vi "Main.vi"(9 "Marca":T1, 10 "Com Port":refnum<visa-resource-name>, 11 "Module Admin":refnum<class "Delacor_lib_QMH_Cloneable Module Admin.lvclass">) -> ()   [LabVIEW 2019, in "Multiple_uC.lvlib"]
doc: "This template is based off of the Queued Message Handler design pattern and the Queued Message Handler project template that ships with LabVIEW.\n\nThe main difference is that the queue is private to this module and communication between modules is performed via Broadcast and Request events.\n\nRequest events are wrapped in public API methods and are handled in the Event Handling Loop (EHL) of this VI. Any module can register for Broadcast events sent by this module. The EHL generates messages based on user interface actions.\n\nThe Message Handling Loop (MHL) processes messages generated by the EHL, or by other messages. The messages are string values, so new messages can be added easily to the Message Cases case structure in the MHL. Each message cluster can also provide an optional value for Message Data, which is a variant that can be converted to whatever message-specific data is required.\n_____\nBased on Delacor QMH Project Template 5.0.0.82."
uses:
  Multiple_uC.lvlib
  <vilib>/Delacor/Delacor QMH/Libraries/Cloneable Module Admin_class/Delacor_lib_QMH_Cloneable Module Admin.lvclass
  C:/Program Files/National Instruments/LabVIEW 2019/vi.lib/Delacor/Delacor QMH/Libraries/Module Admin_class/Delacor_lib_QMH_Module Admin.lvclass
  Clase Padre/Marca.ctl
  Module Data--cluster.ctl
  Clase Padre/Serial Device.lvclass
  <vilib>/Delacor/Delacor QMH/Libraries/Message Queue_class/Delacor_lib_QMH_Message Queue.lvclass/Delacor_lib_QMH_Message Queue.ctl
  <vilib>/Delacor/Delacor QMH/Libraries/Cloneable Module Admin_class/Delacor_lib_QMH_Cloneable Module Admin.lvclass/Delacor_lib_QMH_Cloneable Module Admin.ctl
  Stop Argument--cluster.ctl
  <vilib>/Delacor/Delacor QMH/Libraries/Module Admin_class/Delacor_lib_QMH_Module Admin.lvclass/Delacor_lib_QMH_Module Admin.ctl
  Write_1BIT Argument--cluster.ctl
  Write_1BIT (Reply Payload)--cluster.ctl
  Set 8 bits Argument--cluster.ctl
  Set 8 bits (Reply Payload)--cluster.ctl
  GET_1BIT Argument--cluster.ctl
  GET_1BIT (Reply Payload)--cluster.ctl
  GET_8BITS Argument--cluster.ctl
  GET_8BITS (Reply Payload)--cluster.ctl
  <vilib>/Utility/miscctls.llb/LVPointTypeDef.ctl
  Clases Hijos/NXP/NXP.lvclass
  C:/Users/Luis/Documents/Ingenieria/Git_versiones/PROYECTO-FINAL-INSTRUMENTACI-N-VIRTUAL/Clase Padre/Serial Device.lvclass
  Clases Hijos/Simulated/Simulated uC.lvclass
  Clases Hijos/Cypress/Cypress.lvclass
  Clase Padre/Serial Device.lvclass/Serial Device.ctl
  <vilib>/Delacor/Delacor QMH/Libraries/Message Queue_class/Delacor_lib_QMH_Enqueue Message (Single).vi
  <vilib>/Delacor/Delacor QMH/Libraries/Cloneable Module Admin_class/Delacor_lib_QMH_Get Module ID.vi
  <vilib>/Delacor/Delacor QMH/Libraries/Module Admin_class/Delacor_lib_QMH_Get External Launch.vi
  <vilib>/Utility/error.llb/Error Cluster From Error Code.vi
  <vilib>/ErrorRing/Error Ring.xnode
  <vilib>/Delacor/Delacor QMH/Libraries/Message Queue_class/Delacor_lib_QMH_Message Queue.lvclass
panel:
  in  "Read\n8 BITS":bool
  out "Response R 8BIT":string
  out "Response R 1BIT":string
  in  "GET 1BIT":u8 max=7
  out "Response W 8_B":string
  in  "Number":u8
  out "Response W1BIT":string
  in  "Encender\n W1BIT?":bool
  in  "Bit W1BIT":u8 max=7
  out "Response ADC":string
  in  "Channel adc":u8 max=9
  in  "Simulate MHL Error":bool
  in  "Simulate EHL Error":bool
  out "error out":errorcluster
  out "Status":string
  # "ADC"
  # "Write 1 Bit"
  # "Write 8 bit"
  # "Read 1 Bit"
  # "Read 8 bits"
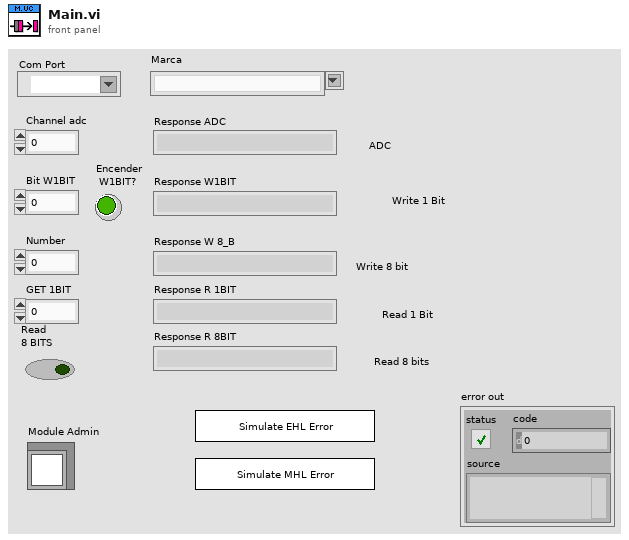
[diagram p1: front panel]
types:
  T1 = typedef "Marca.ctl" = string
  T2 = typedef "Multiple_uC.lvlib/Request Events--cluster.ctl" = cluster{"Stop Module":refnum<user-event>, "Show Panel":refnum<user-event>, "Hide Panel":refnum<user-event>, "Show Diagram":refnum<user-event>, "Get Module Execution Status":refnum<user-event>, "ADC´s View":refnum<user-event>, "Write_1BIT":refnum<user-event>, "Set 8 bits":refnum<user-event>, "GET_1BIT":refnum<user-event>, "GET_8BITS":refnum<user-event>}
  T3 = typedef "Multiple_uC.lvlib/Module Data--cluster.ctl" = cluster{"Status":string, "Serial Device.lvclass":refnum<class "Serial Device.lvclass">}
  T4 = enum32{"invalid lock state", "Not Locked", "Locked (No Password)", "Password-protected"}
  T5 = typedef "Multiple_uC.lvlib/Stop Argument--cluster.ctl" = cluster{"Module ID":i32, "Origin":string, "Exit via Stop Module Req?":bool, "Wait for Module to stop?":bool}
  T6 = typedef "Multiple_uC.lvlib/ADC´s View Argument--cluster.ctl" = cluster{"Module ID":i32, "Channel":u8, "Wait Notifier":refnum<notifier>, "wait for reply":bool}
  T7 = typedef "Multiple_uC.lvlib/Write_1BIT Argument--cluster.ctl" = cluster{"Module ID":i32, "Channel":u8, "Encender?":bool, "Wait Notifier":refnum<notifier>, "wait for reply":bool}
  T8 = typedef "Multiple_uC.lvlib/Set 8 bits Argument--cluster.ctl" = cluster{"Module ID":i32, "Number":u8, "Wait Notifier":refnum<notifier>, "wait for reply":bool}
  T9 = typedef "Multiple_uC.lvlib/GET_1BIT Argument--cluster.ctl" = cluster{"Module ID":i32, "GET 1BIT":u8, "Wait Notifier":refnum<notifier>, "wait for reply":bool}
  T10 = typedef "Multiple_uC.lvlib/GET_8BITS Argument--cluster.ctl" = cluster{"Module ID":i32, "Wait Notifier":refnum<notifier>, "wait for reply":bool, "Canal":u8}
  T11 = typedef "LVPointTypeDef.ctl" = cluster{"Horizontal":i16, "Vertical":i16}
  T12 = enum32{"Invalid", "Standard", "Closed", "Hidden", "Minimized", "Maximized"}
  T13 = typedef "Multiple_uC.lvlib/ADC´s View (Reply Payload)--cluster.ctl" = cluster{"Expected Response":string, "Numeric":dbl, "ADC´s View_error":errorcluster}
  T14 = typedef "Multiple_uC.lvlib/Write_1BIT (Reply Payload)--cluster.ctl" = cluster{"Response Write_1B":string, "Write_1BIT_error":errorcluster}
  T15 = typedef "Multiple_uC.lvlib/Set 8 bits (Reply Payload)--cluster.ctl" = cluster{"Response":string, "Set 8 bits_error":errorcluster}
  T16 = typedef "Multiple_uC.lvlib/GET_1BIT (Reply Payload)--cluster.ctl" = cluster{"Response 1BIT":string, "GET_1BIT_error":errorcluster}
  T17 = typedef "Multiple_uC.lvlib/GET_8BITS (Reply Payload)--cluster.ctl" = cluster{"Response 8Bits":string, "GET_8BITS_error":errorcluster}
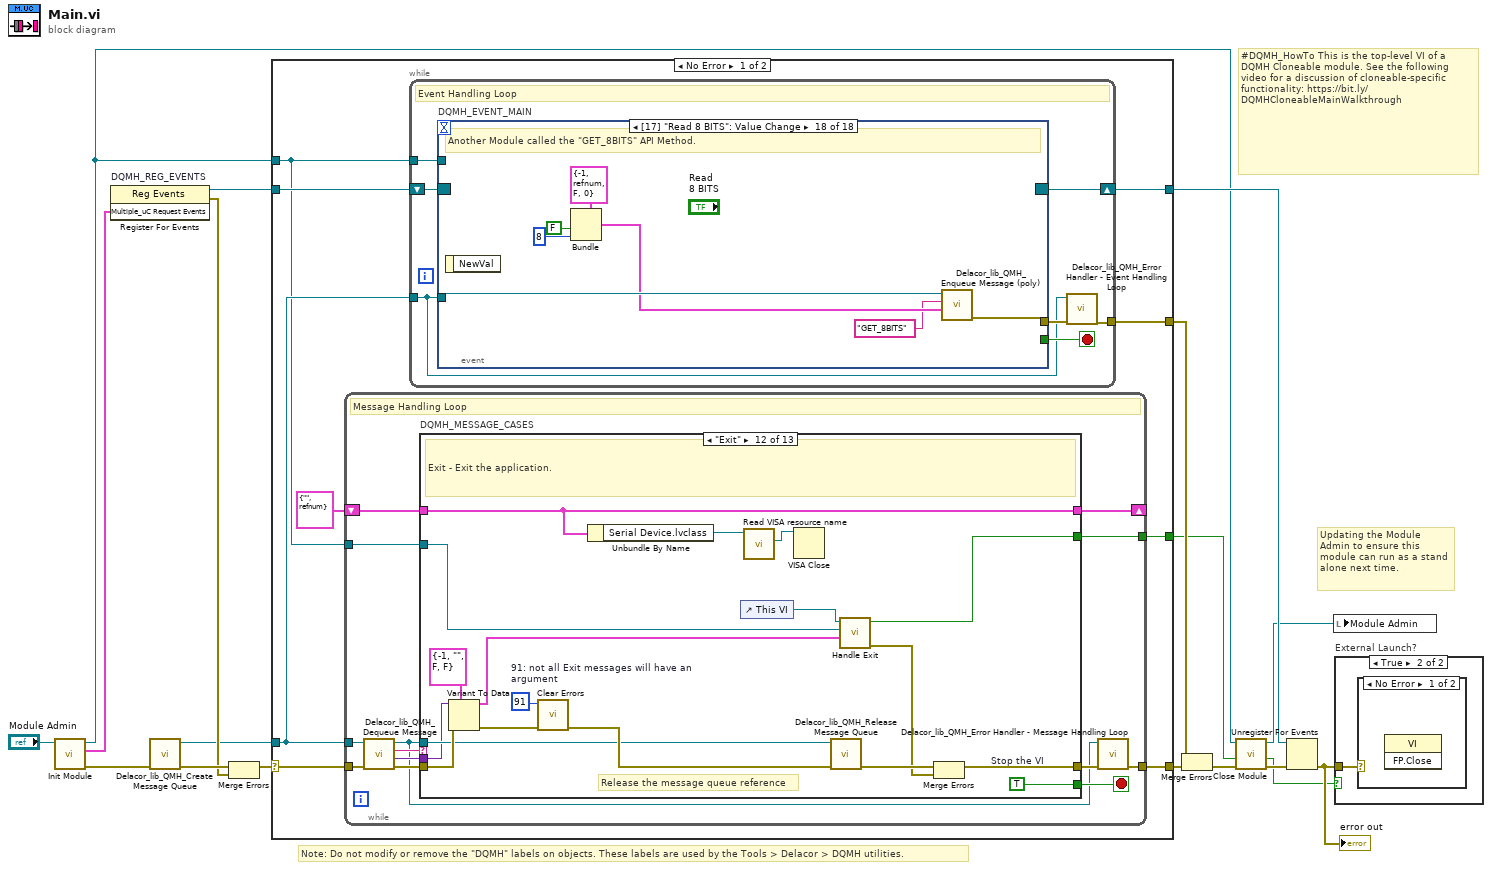
[diagram p0: block diagram]
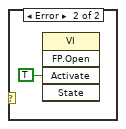
[diagram p3: hidden frame]
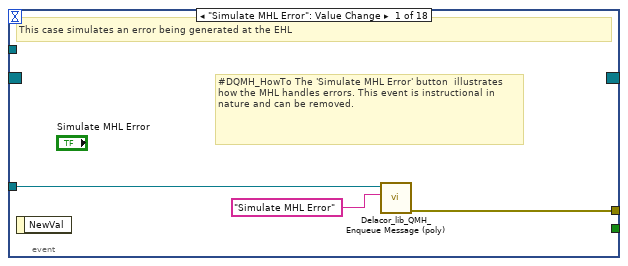
[diagram p4: hidden frame]
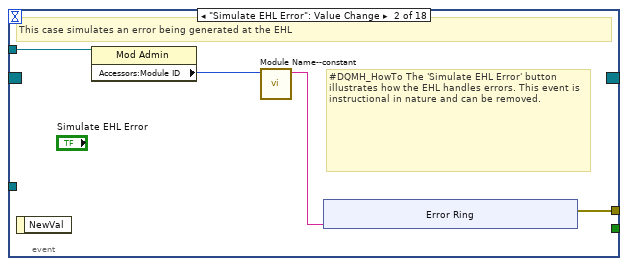
[diagram p5: hidden frame]
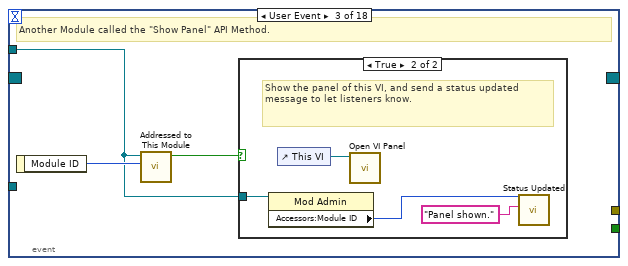
[diagram p6: hidden frame]
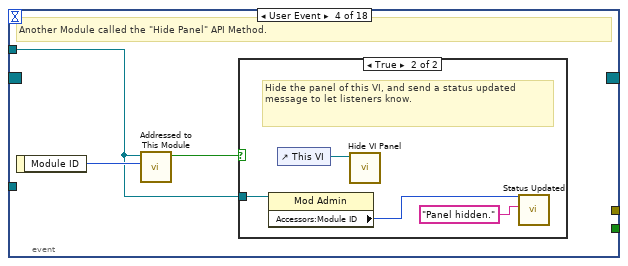
[diagram p8: hidden frame]
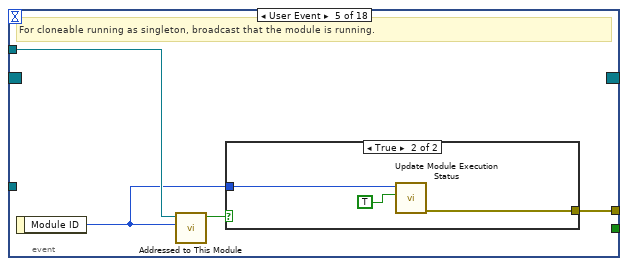
[diagram p10: hidden frame]
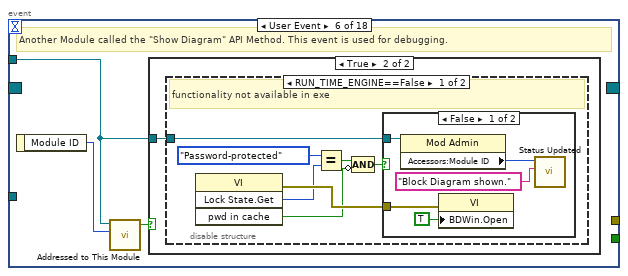
[diagram p12: hidden frame]
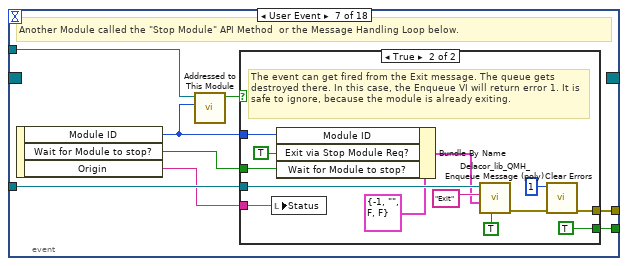
[diagram p16: hidden frame]
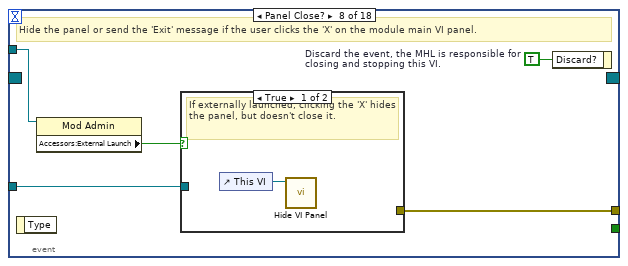
[diagram p18: hidden frame]
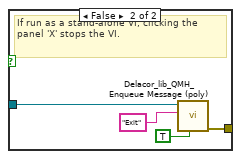
[diagram p19: hidden frame]
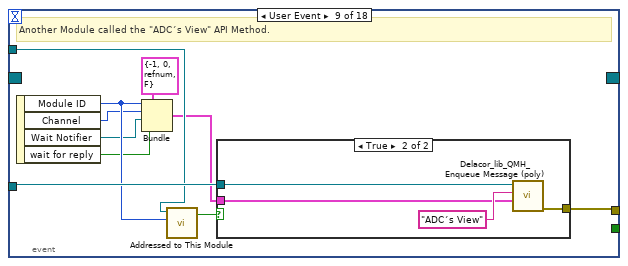
[diagram p20: hidden frame]
diagram:
  # "#DQMH_HowTo This is the top-level VI of a DQMH Cloneable module. See the following video for a discussion of cloneable-specific functionality: https://bit.ly/DQMHCloneableMainWalkthrough"
  # "Note: Do not modify or remove the \"DQMH\" labels on objects. These labels are used by the Tools > Delacor > DQMH utilities."
  # "Updating the Module Admin to ensure this module can run as a stand alone next time."
  n1 = call "Init Module.vi"("Cloneable Module Admin in"="Module Admin") -> ("error out"=w15:errorcluster, "Multiple_uC Request Events"=w7:T2, "Cloneable Module Admin out"=w4:refnum<class "Delacor_lib_QMH_Cloneable Module Admin.lvclass">)  [unwired: 8 in]
  n2 = register-events "DQMH_REG_EVENTS"(w7) -> (reference out=w8:refnum<event-registration>, error out=w10:errorcluster)  [unwired: 2 in]
  n3 = call <vilib>:"Delacor_lib_QMH_Create Message Queue.vi"("error in (no error)"=w15) -> ("error out"=w12:errorcluster, "Message Queue"=w6:refnum<class "Delacor_lib_QMH_Message Queue.lvclass">)  [unwired: 9 in]
  n4 = Merge Errors(w12, w10) -> (w11:errorcluster)
  n5 = case shown="No Error" w11 {
    selector: w11 -> [w25 w445]
    tunnel: [w27 w444] -> w16
    tunnel: [w24 w452] -> w9
    tunnel: w8 -> [w22 w452]
    tunnel: w6 -> [w21 w443]
    tunnel: [w26 _] -> w17
    tunnel: w4 -> [w20 w448]
    tunnel: [w19 _] -> w2
    frame No Error {
      n6 = while {
        tunnel: w21 -> [w227]
        shift-right: [w231] -> _
        shift-left: T3 {"Status"="", "Serial Device.lvclass"=refnum} ("Data Cluster") -> [w232]
        tunnel: w25 -> [w235]
        tunnel: [w233] -> w27
        tunnel: w20 -> [w225]
        tunnel: [w224] -> w19
        stop <- w230 stop-if-true
        # "Message Handling Loop"
        n7 = call-dynamic "Delacor_lib_QMH_Dequeue Message.vi"("error in (no error)"=w235, "Message Queue in"=w227) -> ("error out"=w234:errorcluster, "Message Data"=w228:variant, "Message"=w229:string, "Message Queue out"=w226:refnum<class "Delacor_lib_QMH_Message Queue.lvclass">)  [unwired: 6 in]
        n8 = case "DQMH_MESSAGE_CASES" shown="\"Exit\"" w229 {
          selector: w229 -> [_ _ _ _ _ _ _ _ _ _ _ _ w430]
          tunnel: w226 -> [_ _ _ _ _ _ _ _ _ w368 _ w420 _]
          tunnel: w234 -> [w262 w272 w288 w306 w323 w340 w357 w362 w364 w376 w401 w426 w432]
          tunnel: [w260 w272 w279 w297 w314 w331 w348 w361 w364 w372 w400 w423 w433] -> w236
          tunnel: w232 -> [w253 w271 w278 w296 w313 w330 w347 w360 w363 w365 w398 w410 w431]
          tunnel: [w252 w271 w278 w296 w313 w330 w347 w360 w363 w365 w398 w410 w431] -> w231
          tunnel: [_ _ _ _ _ _ _ _ _ _ _ w419 _] -> w230
          tunnel: w228 -> [_ _ w286 w304 w321 w338 w355 _ _ w371 _ w417 _]
          tunnel: w225 -> [w247 _ _ _ _ _ _ _ _ w370 w396 w413 w428]
          tunnel: [_ _ _ _ _ _ _ _ _ _ _ w415 _] -> w224
          frame "Initialize" {
            w244 = "Initial Message" ("Initial Message")
            # "Initialize - Any operation that needs to be done before the module can receive messages. Synchronize Caller Events.vi will inform Start Module.vi that the module has launched and is ready to receive messages. Module Did Init.vi will broadcast that the module initialized."
            n9 = call "Synchronize Caller Events.vi"("error in (no error)"=w262, "Module Admin"=w247) -> ("error out"=w261:errorcluster, "Module Admin out"=w246:refnum<class "Delacor_lib_QMH_Cloneable Module Admin.lvclass">)  [unwired: 8 in]
            n10 = property class="Mod Admin"(reference=w246) -> ("Accessors:Module ID"=w249:i32, "Accessors:External Launch"=w248:bool)  [unwired: 1 in, 2 out]
            n11 = case shown="\"N\", Default" "Marca" {
              tunnel: [refnum<class "NXP.lvclass"> refnum ("NXP.lvclass") refnum<class "Simulated uC.lvclass"> refnum ("Simulated uC.lvclass") refnum<class "Cypress.lvclass"> refnum ("Cypress.lvclass")] -> w243
              frame "N", Default {
                n12 = One Button Dialog(message="NXP") -> ()  [unwired: 1 in, 1 out]
              }
              frame "S" {
                n13 = One Button Dialog(message="Sim") -> ()  [unwired: 1 in, 1 out]
              }
              frame "C" {
                n14 = One Button Dialog(message="Cypress") -> ()  [unwired: 1 in, 1 out]
              }
            }
            n15 = call "Module Name--constant.vi"("Module ID"=w249) -> ("Module Name"=w257:string)  [unwired: 10 in]
            n16 = VISA Open(VISA resource name="Com Port") -> (VISA resource name=w238:refnum<visa-resource-name>)  [unwired: 4 in, 1 out]
            n17 = call "Write Marca.vi"("Marca"="Marca", "Serial Device in"=w243) -> ("Serial Device out"=w242:refnum<class "Serial Device.lvclass">)  [unwired: 8 in, 1 out]
            n18 = call "Write VISA resource name.vi"("VISA resource name"=w238, "Serial Device in"=w242) -> ("Serial Device out"=w240:refnum<class "Serial Device.lvclass">)  [unwired: 8 in, 1 out]
            n19 = property class="VI"("Front Panel.Title"=w257) -> (reference out=w259:refnum<vi>, error out=w264:errorcluster)  [unwired: 2 in]
            n20 = Select(t=T12."Hidden" ("State"), s=w248, f=T12."Standard" ("State")) -> (s? t:f=w254:T12)
            n21 = call-dynamic "Initialize.vi"("Serial Device in"=w240) -> ("Serial Device out"=w239:refnum<class "Serial Device.lvclass">)  [unwired: 9 in, 1 out]
            n22 = Bundle By Name(cluster=w253, "Serial Device.lvclass"=w239, "Status"=w244) -> (w252:T3)
            n23 = invoke class="VI" method="FP.Open"(reference=w259, error in=w264, "State"=w254) -> (reference out=w258:refnum<vi>, error out=w263:errorcluster)  [unwired: 2 in, 3 out]
            n24 = call "Module Name--constant.vi"("Module ID"=w249) -> ("Module Name"=w250:string)  [unwired: 10 in]
            n25 = invoke class="VI" method="FP.Center"(reference=w258, error in=w263) -> ()  [unwired: 1 in, 3 out]
            n26 = property on="Pane" class="Pane"("Origin"=T11 {"Horizontal"=0, "Vertical"=0}) -> ()  [unwired: 2 in, 2 out]
            n27 = call "Module Did Init.vi"("error in (no error)"=w261, "Initialized?"=TRUE, "Origin"=w250, "Module ID"=w249) -> ("error out"=w260:errorcluster)  [unwired: 7 in]
            "Status" <- w244
          }
          frame "--- Module Specific ---" {
            # "Separator -- The following cases handle messages specific to this Module."
          }
          frame "ADC´s View" {
            # "Request and wait for reply of ADC Channel"
            n28 = Unbundle By Name(w278) -> ("Serial Device.lvclass"=w277:refnum<class "Serial Device.lvclass">)
            n29 = Variant To Data(error in=w288, type=T6 {"Module ID"=-1, "Channel"=0, "Wait Notifier"=refnum, "wait for reply"=FALSE} ("ADC´s View Argument"), Variant=w286) -> (data=w284:T6, error out=w287:errorcluster)
            n30 = Unbundle By Name(w284) -> ("Channel"=w276:u8, "Wait Notifier"=w283:refnum<notifier>, "wait for reply"=w282:bool)
            n31 = call-dynamic "Send_ADC.vi"("Channel"=w276, "Serial Device in"=w277) -> ("error out"=w273:errorcluster, "Response"=w274:string)  [unwired: 7 in, 1 out]
            "Response ADC" <- w274
            n32 = Decimal String To Number(string=w274) -> (offset past number=w275:i32)  [unwired: 2 in, 1 out]
            n33 = Bundle By Name(cluster=T13 {"Expected Response"="", "Numeric"=0.0, "ADC´s View_error"={"status"=FALSE, "code"=0, "source"=""}} ("ADC´s View (Reply Payload)"), "Expected Response"=w274, "Numeric"=w275, "ADC´s View_error"=w273) -> (w281:T13)
            n34 = case shown="True" w282 {
              tunnel: w283 -> [_ w290]
              tunnel: w281 -> [_ w289]
              frame False {
              }
              frame True {
                n35 = Send Notification(notification=w289, notifier=w290) -> ()  [unwired: 1 in, 2 out]
              }
            }
            n36 = Merge Errors(w287, w273) -> (w279:errorcluster)
          }
          frame "Write_1BIT" {
            # "Event to rewrite the value of one bit in an array"
            n37 = Unbundle By Name(w296) -> ("Serial Device.lvclass"=w295:refnum<class "Serial Device.lvclass">)
            n38 = Variant To Data(error in=w306, type=T7 {"Module ID"=-1, "Channel"=0, "Encender?"=FALSE, "Wait Notifier"=refnum, "wait for reply"=FALSE} ("Write_1BIT Argument"), Variant=w304) -> (data=w302:T7, error out=w305:errorcluster)
            n39 = Unbundle By Name(w302) -> ("Channel"=w294:u8, "Encender?"=w293:bool, "Wait Notifier"=w301:refnum<notifier>, "wait for reply"=w300:bool)
            n40 = call-dynamic "Send_SET_1BIT.vi"("Encender?"=w293, "Channel"=w294, "Serial Device in"=w295) -> ("error out"=w291:errorcluster, "Response"=w292:string)  [unwired: 6 in, 1 out]
            "Response W1BIT" <- w292
            n41 = Bundle By Name(cluster=T14 {"Response Write_1B"="", "Write_1BIT_error"={"status"=FALSE, "code"=0, "source"=""}} ("Write_1BIT (Reply Payload)"), "Response Write_1B"=w292, "Write_1BIT_error"=w291) -> (w299:T14)
            n42 = case shown="True" w300 {
              tunnel: w301 -> [_ w308]
              tunnel: w299 -> [_ w307]
              frame False {
              }
              frame True {
                n43 = Send Notification(notification=w307, notifier=w308) -> ()  [unwired: 1 in, 2 out]
              }
            }
            n44 = Merge Errors(w305, w291) -> (w297:errorcluster)
          }
          frame "Set 8 bits" {
            # "Set a number of 8 bits in the microcontroller"
            n45 = Unbundle By Name(w313) -> ("Serial Device.lvclass"=w309:refnum<class "Serial Device.lvclass">)
            n46 = Variant To Data(error in=w323, type=T8 {"Module ID"=-1, "Number"=0, "Wait Notifier"=refnum, "wait for reply"=FALSE} ("Set 8 bits Argument"), Variant=w321) -> (data=w319:T8, error out=w322:errorcluster)
            n47 = Unbundle By Name(w319) -> ("Number"=w312:u8, "Wait Notifier"=w318:refnum<notifier>, "wait for reply"=w317:bool)
            n48 = call-dynamic "Send_SET_8Bits.vi"("Channel"=w312, "Serial Device in"=w309) -> ("error out"=w310:errorcluster, "Response"=w311:string)  [unwired: 7 in, 1 out]
            "Response W 8_B" <- w311
            n49 = Bundle By Name(cluster=T15 {"Response"="", "Set 8 bits_error"={"status"=FALSE, "code"=0, "source"=""}} ("Set 8 bits (Reply Payload)"), "Response"=w311, "Set 8 bits_error"=w310) -> (w316:T15)
            n50 = case shown="False" w317 {
              tunnel: w318 -> [_ w325]
              tunnel: w316 -> [_ w324]
              frame False {
              }
              frame True {
                n51 = Send Notification(notification=w324, notifier=w325) -> ()  [unwired: 1 in, 2 out]
              }
            }
            n52 = Merge Errors(w322, w310) -> (w314:errorcluster)
          }
          frame "GET_1BIT" {
            # "Obtain the value of 1 specific bit of the input of the microcontroller"
            n53 = Unbundle By Name(w330) -> ("Serial Device.lvclass"=w329:refnum<class "Serial Device.lvclass">)
            n54 = Variant To Data(error in=w340, type=T9 {"Module ID"=-1, "GET 1BIT"=0, "Wait Notifier"=refnum, "wait for reply"=FALSE} ("GET_1BIT Argument"), Variant=w338) -> (data=w336:T9, error out=w339:errorcluster)
            n55 = Unbundle By Name(w336) -> ("GET 1BIT"=w328:u8, "Wait Notifier"=w335:refnum<notifier>, "wait for reply"=w334:bool)
            n56 = call-dynamic "Send_Get_1Bit.vi"("Channel"=w328, "Serial Device in"=w329) -> ("error out"=w326:errorcluster, "Response"=w327:string)  [unwired: 7 in, 1 out]
            "Response R 1BIT" <- w327
            n57 = Bundle By Name(cluster=T16 {"Response 1BIT"="", "GET_1BIT_error"={"status"=FALSE, "code"=0, "source"=""}} ("GET_1BIT (Reply Payload)"), "Response 1BIT"=w327, "GET_1BIT_error"=w326) -> (w333:T16)
            n58 = case shown="True" w334 {
              tunnel: w335 -> [_ w342]
              tunnel: w333 -> [_ w341]
              frame False {
              }
              frame True {
                n59 = Send Notification(notification=w341, notifier=w342) -> ()  [unwired: 1 in, 2 out]
              }
            }
            n60 = Merge Errors(w339, w326) -> (w331:errorcluster)
          }
          frame "GET_8BITS" {
            # "Event created to get the eight bits of the eight inputs in the microcontroller"
            n61 = Unbundle By Name(w347) -> ("Serial Device.lvclass"=w346:refnum<class "Serial Device.lvclass">)
            n62 = Variant To Data(error in=w357, type=T10 {"Module ID"=-1, "Wait Notifier"=refnum, "wait for reply"=FALSE, "Canal"=0} ("GET_8BITS Argument"), Variant=w355) -> (data=w353:T10, error out=w356:errorcluster)
            n63 = Unbundle By Name(w353) -> ("Canal"=w345:u8, "Wait Notifier"=w352:refnum<notifier>, "wait for reply"=w351:bool)
            n64 = call-dynamic "Send_Get_8Bits.vi"("Channel"=w345, "Serial Device in"=w346) -> ("error out"=w343:errorcluster, "Response"=w344:string)  [unwired: 7 in, 1 out]
            "Response R 8BIT" <- w344
            n65 = Bundle By Name(cluster=T17 {"Response 8Bits"="", "GET_8BITS_error"={"status"=FALSE, "code"=0, "source"=""}} ("GET_8BITS (Reply Payload)"), "Response 8Bits"=w344, "GET_8BITS_error"=w343) -> (w350:T17)
            n66 = case shown="True" w351 {
              tunnel: w352 -> [_ w359]
              tunnel: w350 -> [_ w358]
              frame False {
              }
              frame True {
                n67 = Send Notification(notification=w358, notifier=w359) -> ()  [unwired: 1 in, 2 out]
              }
            }
            n68 = Merge Errors(w356, w343) -> (w348:errorcluster)
          }
          frame "---Copy This Frame---" {
            # "Duplicate this frame when creating new messages.  Change this comment in the duplicated frame to describe this message."
            n69 = Merge Errors(w362) -> (w361:errorcluster)
          }
          frame "--- Exit and Error Handling---" {
            # "Separator - the following cases handle errors and exit messages."
          }
          frame "Error" {
            # "Error - Check the error message data and respond accordingly. This message is sent by the \"Error Handler\" VIs at the end of each loop in this application."
            n70 = property class="Mod Admin"(reference=w370) -> ("Accessors:External Launch"=w369:bool, "Accessors:Module ID"=w366:i32)  [unwired: 1 in, 2 out]
            n71 = Variant To Data(error in=w376, type=errorcluster {"status"=FALSE, "code"=0, "source"=""} ("error constant"), Variant=w371) -> (data=w377:errorcluster, error out=w374:errorcluster)
            n72 = call "Module Name--constant.vi"("Module ID"=w366) -> ("Module Name"=w367:string)  [unwired: 10 in]
            n73 = call "Error Reported.vi"("Additional Information"=w367, "Error"=w377, "Module ID"=w366) -> ()  [unwired: 8 in, 1 out]
            n74 = case shown="True" w369 {
              tunnel: [w382 w383] -> w373
              tunnel: w368 -> [w380 w384]
              tunnel: w377 -> [w381 w386]
              frame False {
                # "If the module is running standalone, then pop up an error dialog and call the \"Exit\" message."
                n75 = call <vilib>:"Simple Error Handler.vi"("error in (no error)"=w381) -> ()  [unwired: 4 in, 5 out]
                n76 = call-poly <vilib>:"Delacor_lib_QMH_Enqueue Message (poly).vi"("Priority Message? (F)"=TRUE, "Message"="Exit", "Message Queue in"=w380) -> ("error out"=w382:errorcluster)  [unwired: 7 in, 1 out]
              }
              frame True {
                n77 = Unbundle By Name(w386) -> ("code"=w385:i32)
                n78 = case shown="-1073807360" w385 {
                  tunnel: w384 -> [_ w390 w394]
                  tunnel: [_ w387 w391] -> w383
                  frame 0, Default {
                  }
                  frame -1073807360 {
                    n79 = call-poly <vilib>:"Delacor_lib_QMH_Enqueue Message (poly).vi"("Message"="Exit", "Message Queue in"=w390) -> ("error out"=w387:errorcluster)  [unwired: 8 in, 1 out]
                    n80 = One Button Dialog(message="Microcontrolador\nDesconectado\n:(\n\nFavor de revisar la conexión y vuelva a intentar") -> ()  [unwired: 1 in, 1 out]
                  }
                  frame -1073807343 {
                    n81 = One Button Dialog(message="Microcontrolador\nDesconectado\n:(\n\nFavor de revisar la conexión y vuelva a intentar") -> ()  [unwired: 1 in, 1 out]
                    n82 = call-poly <vilib>:"Delacor_lib_QMH_Enqueue Message (poly).vi"("Message"="Exit", "Message Queue in"=w394) -> ("error out"=w391:errorcluster)  [unwired: 8 in, 1 out]
                  }
                }
              }
            }
            n83 = Merge Errors(w374, w373) -> (w372:errorcluster)
            n84 = local write "error out"(w372) -> ()
          }
          frame "Simulate MHL Error" {
            # "#DQMH_HowTo The 'Simulate MHL Error' button  illustrates how the MHL handles errors. This event is instructional in nature and can be removed."
            # "Simulate an error occurring at the MHL"
            n85 = property class="Mod Admin"(reference=w396) -> ("Accessors:Module ID"=w397:i32)  [unwired: 1 in, 2 out]
            n86 = call "Module Name--constant.vi"("Module ID"=w397) -> ("Module Name"=w395:string)  [unwired: 10 in]
            n87 = xnode "Error Ring"("parameter 0"=w395) -> ("error out"=w399:errorcluster)
            n88 = Merge Errors(w401, w399) -> (w400:errorcluster)
          }
          frame "Exit" {
            w418 = 91  # 91: not all Exit messages will have an argument
            w419 = TRUE  # Stop the VI
            # "Release the message queue reference"
            # "Exit - Exit the application."
            n89 = Variant To Data(error in=w426, type=T5 {"Module ID"=-1, "Origin"="", "Exit via Stop Module Req?"=FALSE, "Wait for Module to stop?"=FALSE} ("Stop Argument"), Variant=w417) -> (data=w414:T5, error out=w421:errorcluster)
            n90 = call <vilib>:"Clear Errors.vi"("error in (no error)"=w421, "specific error code to clear (0: all)"=w418) -> ("error out"=w425:errorcluster)  [unwired: 4 in, 1 out]
            n91 = Unbundle By Name(w410) -> ("Serial Device.lvclass"=w409:refnum<class "Serial Device.lvclass">)
            n92 = control-ref of="This VI"() -> (w412:refnum<vi>)
            n93 = call "Read VISA resource name.vi"("Serial Device in"=w409) -> ("VISA resource name"=w411:refnum<visa-resource-name>)  [unwired: 8 in, 2 out]
            n94 = VISA Close(VISA resource name=w411) -> ()  [unwired: 1 in, 1 out]
            n95 = call-dynamic "Delacor_lib_QMH_Release Message Queue.vi"("error in (no error)"=w425, "Message Queue"=w420) -> ("error out"=w424:errorcluster)  [unwired: 9 in]
            n96 = call "Handle Exit.vi"("Stop Argument"=w414, "Module Admin in"=w413, "VI reference"=w412) -> ("error out"=w422:errorcluster, "Wait for Stop?"=w415:bool)  [unwired: 7 in]
            n97 = Merge Errors(w424, w422) -> (w423:errorcluster)
          }
          frame Default {
            # "'Default' case only runs if there is a message that isn't defined in any of the other cases.  Output a programming error."
            n98 = property class="Mod Admin"(reference=w428) -> ("Accessors:Module ID"=w427:i32)  [unwired: 1 in, 2 out]
            n99 = call "Module Name--constant.vi"("Module ID"=w427) -> ("Module Name"=w429:string)  [unwired: 10 in]
            n100 = xnode "Error Ring"("parameter 0"=w430, "parameter 1"=w429) -> ("error out"=w434:errorcluster)
            n101 = Merge Errors(w432, w434) -> (w433:errorcluster)
          }
        }
        n102 = call-dynamic "Delacor_lib_QMH_Error Handler - Message Handling Loop.vi"("error in (no error)"=w236, "Message Queue in"=w226) -> ("dup error in"=w233:errorcluster)  [unwired: 8 in, 1 out]
      }
      n103 = while {
        tunnel: w21 -> [w28]
        shift-right: [w31] -> w24
        shift-left: w22 -> [w32]
        tunnel: [w33] -> w26
        tunnel: w20 -> [w29]
        stop <- w30 stop-if-true
        # "Event Handling Loop"
        n104 = event "DQMH_EVENT_MAIN" shown="[17] \"Read 8 BITS\": Value Change" {
          selector: w32 -> [_ _ _ _ _ _ _ _ _ _ _ _ _ _ _ _ _ _]
          dyn-events: [_ _ _ _ _ _ _ _ _ _ _ _ _ _ _ _ _ _] -> w31
          timeout: _ -> [_ _ _ _ _ _ _ _ _ _ _ _ _ _ _ _ _ _]
          tunnel: [_ _ _ _ _ _ w89 _ _ _ _ _ _ _ _ _ _ _] -> w30
          tunnel: w28 -> [w36 _ _ _ _ _ w92 w108 w126 w137 w148 w160 w170 w181 w191 w202 w212 w223]
          tunnel: [w37 w41 _ _ w66 _ w93 w111 w117 w134 w138 w157 w161 w178 w182 w199 w206 w220] -> w34
          tunnel: w29 -> [_ w40 w49 w56 w64 w70 w91 w109 w124 _ w146 _ w168 _ w189 _ w210 _]
          event "Simulate MHL Error": Value Change {
            # "#DQMH_HowTo The 'Simulate MHL Error' button  illustrates how the MHL handles errors. This event is instructional in nature and can be removed."
            # "This case simulates an error being generated at the EHL"
            n105 = event-data() -> ()  [unwired: 1 in, 1 out]
            n106 = call-poly <vilib>:"Delacor_lib_QMH_Enqueue Message (poly).vi"("Message"="Simulate MHL Error", "Message Queue in"=w36) -> ("error out"=w37:errorcluster)  [unwired: 8 in, 1 out]
          }
          event "Simulate EHL Error": Value Change {
            # "#DQMH_HowTo The 'Simulate EHL Error' button  illustrates how the EHL handles errors. This event is instructional in nature and can be removed."
            # "This case simulates an error being generated at the EHL"
            n107 = event-data() -> ()  [unwired: 1 in, 1 out]
            n108 = property class="Mod Admin"(reference=w40) -> ("Accessors:Module ID"=w39:i32)  [unwired: 1 in, 2 out]
            n109 = call "Module Name--constant.vi"("Module ID"=w39) -> ("Module Name"=w38:string)  [unwired: 10 in]
            n110 = xnode "Error Ring"("parameter 0"=w38) -> ("error out"=w41:errorcluster)
          }
          event User Event {
            # "Another Module called the \"Show Panel\" API Method."
            n111 = event-data() -> ("Module ID"=w50:i32)  [unwired: 1 in]
            n112 = call "Addressed to This Module.vi"("Module ID from Argument"=w50, "Module Admin"=w49) -> ("Addressed to this instance?"=w51:bool)  [unwired: 8 in, 1 out]
            n113 = case shown="True" w51 {
              tunnel: w49 -> [_ w53]
              frame False {
              }
              frame True {
                # "Show the panel of this VI, and send a status updated message to let listeners know."
                n114 = property class="Mod Admin"(reference=w53) -> ("Accessors:Module ID"=w52:i32)  [unwired: 1 in, 2 out]
                n115 = control-ref of="This VI"() -> (w55:refnum<vi>)
                n116 = call "Open VI Panel.vi"("VI"=w55) -> ()  [unwired: 10 in, 1 out]
                n117 = call "Status Updated.vi"("Status"="Panel shown." ("format string"), "Module ID"=w52) -> ()  [unwired: 9 in, 1 out]
              }
            }
          }
          event User Event {
            # "Another Module called the \"Hide Panel\" API Method."
            n118 = event-data() -> ("Module ID"=w57:i32)  [unwired: 1 in]
            n119 = call "Addressed to This Module.vi"("Module ID from Argument"=w57, "Module Admin"=w56) -> ("Addressed to this instance?"=w58:bool)  [unwired: 8 in, 1 out]
            n120 = case shown="True" w58 {
              tunnel: w56 -> [_ w60]
              frame False {
              }
              frame True {
                # "Hide the panel of this VI, and send a status updated message to let listeners know."
                n121 = property class="Mod Admin"(reference=w60) -> ("Accessors:Module ID"=w59:i32)  [unwired: 1 in, 2 out]
                n122 = control-ref of="This VI"() -> (w62:refnum<vi>)
                n123 = call "Hide VI Panel.vi"("VI"=w62) -> ()  [unwired: 10 in, 1 out]
                n124 = call "Status Updated.vi"("Status"="Panel hidden." ("format string"), "Module ID"=w59) -> ()  [unwired: 9 in, 1 out]
              }
            }
          }
          event User Event {
            # "For cloneable running as singleton, broadcast that the module is running."
            n125 = event-data() -> ("Module ID"=w63:i32)  [unwired: 1 in]
            n126 = call "Addressed to This Module.vi"("Module ID from Argument"=w63, "Module Admin"=w64) -> ("Addressed to this instance?"=w65:bool)  [unwired: 8 in, 1 out]
            n127 = case shown="True" w65 {
              tunnel: [_ w69] -> w66
              tunnel: w63 -> [_ w68]
              frame False {
              }
              frame True {
                n128 = call "Update Module Execution Status.vi"("Running?"=TRUE, "Module ID"=w68) -> ("error out"=w69:errorcluster)  [unwired: 9 in]
              }
            }
          }
          event User Event {
            # "Another Module called the \"Show Diagram\" API Method. This event is used for debugging."
            n129 = event-data() -> ("Module ID"=w71:i32)  [unwired: 1 in]
            n130 = call "Addressed to This Module.vi"("Module ID from Argument"=w71, "Module Admin"=w70) -> ("Addressed to this instance?"=w72:bool)  [unwired: 8 in, 1 out]
            n131 = case shown="True" w72 {
              tunnel: w70 -> [_ w73]
              frame False {
              }
              frame True {
                n132 = disable-structure shown="RUN_TIME_ENGINE==False" {
                  disable-tunnel: w73 -> [w74 _]
                  frame condition #0 (active) {
                    # "functionality not available in exe"
                    n133 = invoke class="VI" method="Lock State.Get"() -> (error out=w80:errorcluster, "Get Lock State"=w79:T4, "pwd in cache"=w76:bool)  [unwired: 4 in, 1 out]
                    n134 = Equal?(x=T4."Password-protected", y=w79) -> (x = y?=w77:bool)
                    n135 = Compound Arithmetic op=AND(w77, invert w76) -> (w75:bool)
                    n136 = case shown="False" w75 {
                      tunnel: w80 -> [w85 _]
                      tunnel: w74 -> [w82 _]
                      frame False {
                        n137 = property class="Mod Admin"(reference=w82) -> ("Accessors:Module ID"=w81:i32)  [unwired: 1 in, 2 out]
                        n138 = property class="VI"(error in=w85, "BDWin.Open"=TRUE ("Block Diagram Window:Open")) -> ()  [unwired: 1 in, 2 out]
                        n139 = call "Status Updated.vi"("Status"="Block Diagram shown." ("format string"), "Module ID"=w81) -> ()  [unwired: 9 in, 1 out]
                      }
                      frame True {
                        # "Password-protected VI, and the password is not in the cache. Do not show the diagram."
                      }
                    }
                  }
                  frame condition #1 {
                  }
                }
              }
            }
          }
          event User Event {
            # "Another Module called the \"Stop Module\" API Method  or the Message Handling Loop below."
            n140 = event-data() -> ("Module ID"=w87:i32, "Wait for Module to stop?"=w88:bool, "Origin"=w86:string)  [unwired: 1 in]
            n141 = call "Addressed to This Module.vi"("Module ID from Argument"=w87, "Module Admin"=w91) -> ("Addressed to this instance?"=w90:bool)  [unwired: 8 in, 1 out]
            n142 = case shown="True" w90 {
              tunnel: [_ w105] -> w93
              tunnel: w92 -> [_ w101]
              tunnel: [_ TRUE] -> w89
              tunnel: w88 -> [_ w96]
              tunnel: w87 -> [_ w98]
              tunnel: w86 -> [_ w94]
              frame False {
              }
              frame True {
                # "The event can get fired from the Exit message. The queue gets destroyed there. In this case, the Enqueue VI will return error 1. It is safe to ignore, because the module is already exiting."
                n143 = local write "Status"(w94) -> ()
                n144 = Bundle By Name(cluster=T5 {"Module ID"=-1, "Origin"="", "Exit via Stop Module Req?"=FALSE, "Wait for Module to stop?"=FALSE} ("Stop Argument"), "Module ID"=w98, "Exit via Stop Module Req?"=TRUE, "Wait for Module to stop?"=w96) -> (w95:T5)
                n145 = call-poly <vilib>:"Delacor_lib_QMH_Enqueue Message (poly).vi"("Priority Message? (F)"=TRUE, "Message Data"=w95, "Message"="Exit", "Message Queue in"=w101) -> ("error out"=w106:errorcluster)  [unwired: 6 in, 1 out]
                n146 = call <vilib>:"Clear Errors.vi"("error in (no error)"=w106, "specific error code to clear (0: all)"=1) -> ("error out"=w105:errorcluster)  [unwired: 4 in, 1 out]
              }
            }
          }
          event Panel Close? {
            w110 = TRUE  # Discard the event, the MHL is responsible for closing and stopping this VI.
            # "Hide the panel or send the 'Exit' message if the user clicks the 'X' on the module main VI panel."
            n147 = event-data() -> ()  [unwired: 1 in, 1 out]
            n148 = property class="Mod Admin"(reference=w109) -> ("Accessors:External Launch"=w107:bool)  [unwired: 1 in, 2 out]
            n149 = case shown="True" w107 {
              tunnel: w108 -> [_ w115]
              tunnel: [_ w116] -> w111
              frame True {
                # "If externally launched, clicking the 'X' hides the panel, but doesn't close it."
                n150 = control-ref of="This VI"() -> (w112:refnum<vi>)
                n151 = call "Hide VI Panel.vi"("VI"=w112) -> ()  [unwired: 10 in, 1 out]
              }
              frame False {
                # "If run as a stand-alone VI, clicking the panel 'X' stops the VI."
                n152 = call-poly <vilib>:"Delacor_lib_QMH_Enqueue Message (poly).vi"("Priority Message? (F)"=TRUE, "Message"="Exit", "Message Queue in"=w115) -> ("error out"=w116:errorcluster)  [unwired: 7 in, 1 out]
              }
            }
            n153 = event-data("Discard?"=w110) -> ()  [unwired: 1 in, 1 out]
          }
          event User Event {
            # "Another Module called the \"ADC´s View\" API Method."
            n154 = event-data() -> ("Module ID"=w121:i32, "Channel"=w120:u8, "Wait Notifier"=w119:refnum<notifier>, "wait for reply"=w118:bool)  [unwired: 1 in]
            n155 = Bundle(cluster=T6 {"Module ID"=-1, "Channel"=0, "Wait Notifier"=refnum, "wait for reply"=FALSE} ("ADC´s View Argument"), "Module ID"=w121, "Channel"=w120, "Wait Notifier"=w119, "wait for reply"=w118) -> (w122:T6)
            n156 = call "Addressed to This Module.vi"("Module ID from Argument"=w121, "Module Admin"=w124) -> ("Addressed to this instance?"=w125:bool)  [unwired: 8 in, 1 out]
            n157 = case shown="True" w125 {
              tunnel: w126 -> [_ w130]
              tunnel: w122 -> [_ w128]
              tunnel: [_ w127] -> w117
              frame False {
              }
              frame True {
                n158 = call-poly <vilib>:"Delacor_lib_QMH_Enqueue Message (poly).vi"("Message Data"=w128, "Message"="ADC´s View", "Message Queue in"=w130) -> ("error out"=w127:errorcluster)  [unwired: 7 in, 1 out]
              }
            }
          }
          event "Channel adc": Value Change {
            # "Local Channel ADC"
            n159 = event-data() -> ()  [unwired: 1 in, 3 out]
            n160 = Bundle(cluster=T6 {"Module ID"=-1, "Channel"=0, "Wait Notifier"=refnum, "wait for reply"=FALSE} ("ADC´s View Argument"), "Channel"="Channel adc", "wait for reply"=FALSE) -> (w135:T6)  [unwired: 2 in]
            n161 = call-poly <vilib>:"Delacor_lib_QMH_Enqueue Message (poly).vi"("Message Data"=w135, "Message"="ADC´s View", "Message Queue in"=w137) -> ("error out"=w134:errorcluster)  [unwired: 7 in, 1 out]
          }
          event User Event {
            # "Another Module called the \"Write_1BIT\" API Method."
            n162 = event-data() -> ("Module ID"=w143:i32, "Channel"=w142:u8, "Encender?"=w141:bool, "Wait Notifier"=w140:refnum<notifier>, "wait for reply"=w139:bool)  [unwired: 1 in]
            n163 = Bundle(cluster=T7 {"Module ID"=-1, "Channel"=0, "Encender?"=FALSE, "Wait Notifier"=refnum, "wait for reply"=FALSE} ("Write_1BIT Argument"), "Module ID"=w143, "Channel"=w142, "Encender?"=w141, "Wait Notifier"=w140, "wait for reply"=w139) -> (w144:T7)
            n164 = call "Addressed to This Module.vi"("Module ID from Argument"=w143, "Module Admin"=w146) -> ("Addressed to this instance?"=w147:bool)  [unwired: 8 in, 1 out]
            n165 = case shown="True" w147 {
              tunnel: w148 -> [_ w152]
              tunnel: w144 -> [_ w150]
              tunnel: [_ w149] -> w138
              frame False {
              }
              frame True {
                n166 = call-poly <vilib>:"Delacor_lib_QMH_Enqueue Message (poly).vi"("Message Data"=w150, "Message"="Write_1BIT", "Message Queue in"=w152) -> ("error out"=w149:errorcluster)  [unwired: 7 in, 1 out]
              }
            }
          }
          event "Bit W1BIT": Value Change {
            # "Another Module called the \"Write_1BIT\" API Method."
            n167 = event-data() -> ()  [unwired: 1 in, 1 out]
            n168 = Bundle(cluster=T7 {"Module ID"=-1, "Channel"=0, "Encender?"=FALSE, "Wait Notifier"=refnum, "wait for reply"=FALSE} ("Write_1BIT Argument"), "Channel"="Bit W1BIT", "Encender?"="Encender\n W1BIT?", "wait for reply"=FALSE) -> (w158:T7)  [unwired: 2 in]
            n169 = call-poly <vilib>:"Delacor_lib_QMH_Enqueue Message (poly).vi"("Message Data"=w158, "Message"="Write_1BIT", "Message Queue in"=w160) -> ("error out"=w157:errorcluster)  [unwired: 7 in, 1 out]
          }
          event User Event {
            # "Another Module called the \"Set 8 bits\" API Method."
            n170 = event-data() -> ("Module ID"=w165:i32, "Number"=w164:u8, "Wait Notifier"=w163:refnum<notifier>, "wait for reply"=w162:bool)  [unwired: 1 in]
            n171 = Bundle(cluster=T8 {"Module ID"=-1, "Number"=0, "Wait Notifier"=refnum, "wait for reply"=FALSE} ("Set 8 bits Argument"), "Module ID"=w165, "Number"=w164, "Wait Notifier"=w163, "wait for reply"=w162) -> (w166:T8)
            n172 = call "Addressed to This Module.vi"("Module ID from Argument"=w165, "Module Admin"=w168) -> ("Addressed to this instance?"=w169:bool)  [unwired: 8 in, 1 out]
            n173 = case shown="True" w169 {
              tunnel: w170 -> [_ w174]
              tunnel: w166 -> [_ w172]
              tunnel: [_ w171] -> w161
              frame False {
              }
              frame True {
                n174 = call-poly <vilib>:"Delacor_lib_QMH_Enqueue Message (poly).vi"("Message Data"=w172, "Message"="Set 8 bits", "Message Queue in"=w174) -> ("error out"=w171:errorcluster)  [unwired: 7 in, 1 out]
              }
            }
          }
          event "Number": Value Change {
            # "Another Module called the \"Set 8 bits\" API Method."
            n175 = event-data() -> ()  [unwired: 1 in, 1 out]
            n176 = Bundle(cluster=T8 {"Module ID"=-1, "Number"=0, "Wait Notifier"=refnum, "wait for reply"=FALSE} ("Set 8 bits Argument"), "Number"="Number", "wait for reply"=FALSE) -> (w179:T8)  [unwired: 2 in]
            n177 = call-poly <vilib>:"Delacor_lib_QMH_Enqueue Message (poly).vi"("Message Data"=w179, "Message"="Set 8 bits", "Message Queue in"=w181) -> ("error out"=w178:errorcluster)  [unwired: 7 in, 1 out]
          }
          event User Event {
            # "Another Module called the \"GET_1BIT\" API Method."
            n178 = event-data() -> ("Module ID"=w186:i32, "GET 1BIT"=w185:u8, "Wait Notifier"=w184:refnum<notifier>, "wait for reply"=w183:bool)  [unwired: 1 in]
            n179 = Bundle(cluster=T9 {"Module ID"=-1, "GET 1BIT"=0, "Wait Notifier"=refnum, "wait for reply"=FALSE} ("GET_1BIT Argument"), "Module ID"=w186, "GET 1BIT"=w185, "Wait Notifier"=w184, "wait for reply"=w183) -> (w187:T9)
            n180 = call "Addressed to This Module.vi"("Module ID from Argument"=w186, "Module Admin"=w189) -> ("Addressed to this instance?"=w190:bool)  [unwired: 8 in, 1 out]
            n181 = case shown="True" w190 {
              tunnel: w191 -> [_ w195]
              tunnel: w187 -> [_ w193]
              tunnel: [_ w192] -> w182
              frame False {
              }
              frame True {
                n182 = call-poly <vilib>:"Delacor_lib_QMH_Enqueue Message (poly).vi"("Message Data"=w193, "Message"="GET_1BIT", "Message Queue in"=w195) -> ("error out"=w192:errorcluster)  [unwired: 7 in, 1 out]
              }
            }
          }
          event "GET 1BIT": Value Change {
            # "Another Module called the \"GET_1BIT\" API Method."
            n183 = event-data() -> ()  [unwired: 1 in, 1 out]
            n184 = Bundle(cluster=T9 {"Module ID"=-1, "GET 1BIT"=0, "Wait Notifier"=refnum, "wait for reply"=FALSE} ("GET_1BIT Argument"), "GET 1BIT"="GET 1BIT", "wait for reply"=FALSE) -> (w200:T9)  [unwired: 2 in]
            n185 = call-poly <vilib>:"Delacor_lib_QMH_Enqueue Message (poly).vi"("Message Data"=w200, "Message"="GET_1BIT", "Message Queue in"=w202) -> ("error out"=w199:errorcluster)  [unwired: 7 in, 1 out]
          }
          event User Event {
            # "Another Module called the \"GET_8BITS\" API Method."
            n186 = event-data() -> ("Module ID"=w207:i32, "Canal"=w203:u8, "Wait Notifier"=w205:refnum<notifier>, "wait for reply"=w204:bool)  [unwired: 1 in]
            n187 = Bundle(cluster=T10 {"Module ID"=-1, "Wait Notifier"=refnum, "wait for reply"=FALSE, "Canal"=0} ("GET_8BITS Argument"), "Module ID"=w207, "Wait Notifier"=w205, "wait for reply"=w204, "Canal"=w203) -> (w208:T10)
            n188 = call "Addressed to This Module.vi"("Module ID from Argument"=w207, "Module Admin"=w210) -> ("Addressed to this instance?"=w211:bool)  [unwired: 8 in, 1 out]
            n189 = case shown="True" w211 {
              tunnel: w212 -> [_ w216]
              tunnel: w208 -> [_ w214]
              tunnel: [_ w213] -> w206
              frame False {
              }
              frame True {
                n190 = call-poly <vilib>:"Delacor_lib_QMH_Enqueue Message (poly).vi"("Message Data"=w214, "Message"="GET_8BITS", "Message Queue in"=w216) -> ("error out"=w213:errorcluster)  [unwired: 7 in, 1 out]
              }
            }
          }
          event "Read\n8 BITS": Value Change {
            # "Another Module called the \"GET_8BITS\" API Method."
            n191 = event-data() -> ()  [unwired: 1 in, 1 out]
            n192 = Bundle(cluster=T10 {"Module ID"=-1, "Wait Notifier"=refnum, "wait for reply"=FALSE, "Canal"=0} ("GET_8BITS Argument"), "wait for reply"=FALSE, "Canal"=u8 8) -> (w221:T10)  [unwired: 2 in]
            n193 = call-poly <vilib>:"Delacor_lib_QMH_Enqueue Message (poly).vi"("Message Data"=w221, "Message"="GET_8BITS", "Message Queue in"=w223) -> ("error out"=w220:errorcluster)  [unwired: 7 in, 1 out]
          }
        }
        n194 = call-dynamic "Delacor_lib_QMH_Error Handler - Event Handling Loop.vi"("error in (no error)"=w34, "Message Queue in"=w28) -> ("dup error in"=w33:errorcluster)  [unwired: 8 in, 1 out]
      }
    }
    frame Error {
      n195 = call "Synchronize Caller Events.vi"("Module Admin"=w448) -> ("Module Admin out"=w447:refnum<class "Delacor_lib_QMH_Cloneable Module Admin.lvclass">)  [unwired: 9 in, 1 out]
      n196 = property class="Mod Admin"(reference=w447) -> ("Accessors:Module ID"=w446:i32)  [unwired: 1 in, 2 out]
      n197 = call-dynamic "Delacor_lib_QMH_Release Message Queue.vi"("error in (no error)"=w445, "Message Queue"=w443) -> ("error out"=w444:errorcluster)  [unwired: 9 in]
      n198 = call "Module Name--constant.vi"("Module ID"=w446) -> ("Module Name"=w451:string)  [unwired: 10 in]
      n199 = Format Into String(format string="An error occurred during initialization. %s is no longer running.", w451) -> (resulting string=w449:string)  [unwired: 2 in, 1 out]
      n200 = call "Error Reported.vi"("Additional Information"=w449, "Error"=w444, "Module ID"=w446) -> ()  [unwired: 8 in, 1 out]
    }
  }
  n201 = Merge Errors(w17, w16) -> (w18:errorcluster)
  n202 = call "Close Module.vi"("error in"=w18, "Wait for stop?"=w2, "Module Admin in"=w4) -> ("error out"=w14:errorcluster, "External Launch"=w1:bool, "Module Admin out"=w3:refnum<class "Delacor_lib_QMH_Cloneable Module Admin.lvclass">)  [unwired: 6 in]
  n203 = Unregister For Events(event registration refnum=w9, error in=w14) -> (error out=w13:errorcluster)
  "error out" <- w13
  n204 = local write "Module Admin"(w3) -> ()
  n205 = case "External Launch?" shown="True" w1 {
    tunnel: w13 -> [_ w453]
    frame False {
    }
    frame True {
      n206 = case shown="No Error" w453 {
        frame No Error {
          n207 = invoke class="VI" method="FP.Close"() -> ()  [unwired: 3 in, 3 out]
        }
        frame Error {
          n208 = invoke class="VI" method="FP.Open"("Activate"=TRUE ("Activate?")) -> ()  [unwired: 4 in, 5 out]
        }
      }
    }
  }
